vi "CRYPIC POP  Message to MainMenu.vi"(11 "nData":i32) -> (1 "cMsgProject":T1)   [LabVIEW 2013]
uses:
  CRYMain Sub Window Global.vi
panel:
  out "nData_Out":i32
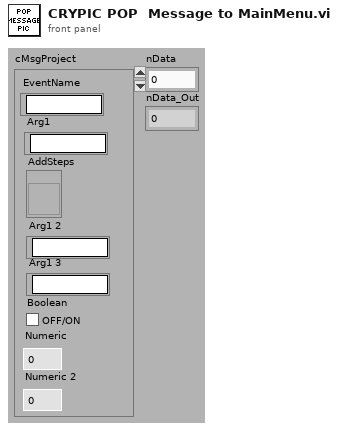
[diagram p1: front panel]
types:
  T1 = cluster{"EventName":string, "Arg1":string, "Numeric":u16, "Numeric 2":u16, "AddSteps ":refnum<vi>, "Arg1 2":string, "Arg1 3":string, "Boolean":bool}
  T2 = cluster{"cMsgProjectList":cluster{"EventName":string, "Arg1":string, "Numeric":u16, "Numeric 2":u16, "AddSteps ":refnum<vi>, "Arg1 2":string, "Arg1 3":string, "Boolean":bool}[], "nIDList":i32[]}
  T3 = cluster{"EventName":string, "Arg1":string, "Numeric":u16, "Numeric 2":u16, "AddSteps ":refnum<vi>, "Arg1 2":string, "Arg1 3":string, "Boolean":bool}[]
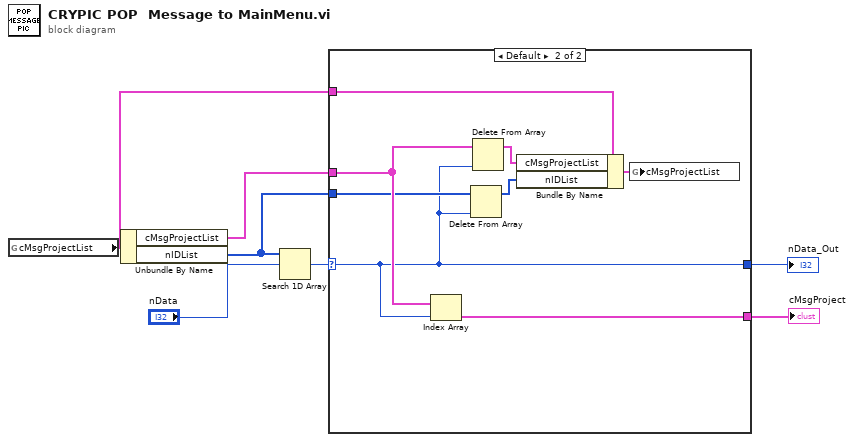
[diagram p0: block diagram]
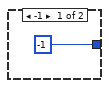
[diagram p2: hidden frame]
diagram:
  n1 = global read "CRYMain Sub Window Global.vi" "cMsgProjectList"() -> (w2:T2)
  n2 = Unbundle By Name(w2) -> ("cMsgProjectList"=w5:T3, "nIDList"=w3:i32[])
  n3 = Search 1D Array(1D array=w3, element="nData") -> (index of element=w7:i32)  [unwired: 1 in]
  n4 = case shown="Default" w7 {
    selector: w7 -> [_ w13]
    tunnel: [-1 ("index of element") w13] -> w6
    tunnel: w5 -> [_ w15]
    tunnel: [_ w16] -> w4
    tunnel: w3 -> [_ w14]
    tunnel: w2 -> [_ w12]
    frame -1 {
    }
    frame Default {
      n5 = Index Array(array=w15, index=w13) -> (element=w16:T1)
      n6 = Delete From Array(array=w14, index=w13) -> (array with subset deleted=w11:i32[])  [unwired: 1 in, 1 out]
      n7 = Delete From Array(array=w15, index=w13) -> (array with subset deleted=w10:T3)  [unwired: 1 in, 1 out]
      n8 = Bundle By Name(cluster=w12, "cMsgProjectList"=w10, "nIDList"=w11) -> (w9:T2)
      n9 = global write "CRYMain Sub Window Global.vi" "cMsgProjectList"(w9) -> ()
    }
  }
  "cMsgProject" <- w4
  "nData_Out" <- w6
